vi "Set Test Method End Time.vi"(11 "LUnit Test Case in":refnum<class "LUnit Test Case.lvclass">) -> (3 "LUnit Test Case out":refnum<class "LUnit Test Case.lvclass">)   [LabVIEW 2020, in "LUnit Test Case.lvclass"]
uses:
  LUnit Test Case.lvclass
  Result Types/Case Result/Test Case Result.lvlib
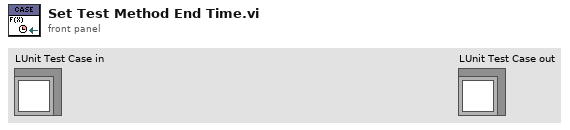
[diagram p1: front panel]
types:
  T1 = typedef "Test Case Result.lvlib/Test Case Result.ctl" = map{string, T2}
  T2 = typedef "Method Result.lvlib/Method Result.ctl" = cluster{"Test Case":string, "Test Method Name":string, "Status":T3, "Assertion Results":T4[], "Execution time":dbl, "Result String":string}
  T3 = typedef "Assertion Result.lvlib/Status.ctl" = enum16{"Pass", "Fail", "Error", "Skipped", "Setup Error", "Broken", "Teardown Error"}
  T4 = typedef "Assertion Result.lvlib/Assertion Result.ctl" = cluster{"Status":T3, "Message":string, "Description":string, "Assertion Type":T5}
  T5 = typedef "Assertion Result.lvlib/Assertion Type.ctl" = enum16{"None", "Pass", "Fail", "Skip", "Pass if Equal", "Fail if Equal", "Pass if Error", "Fail if Error", "Pass if", "Fail if"}
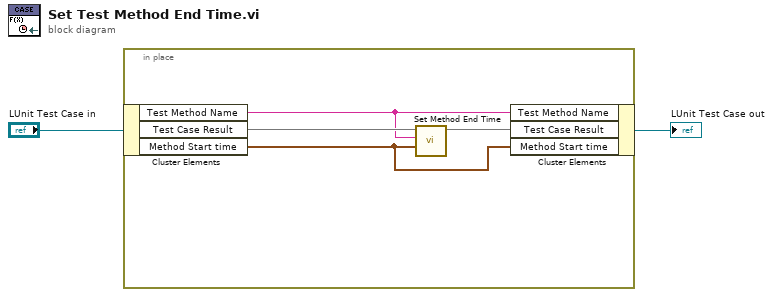
[diagram p0: block diagram]
diagram:
  n1 = in-place {
    n2 = in-place-cluster #1("LUnit Test Case in") -> ("Test Method Name"=w4:string, "Test Case Result"=w6:T1, "Method Start time"=w3:timestamp)
    n3 = call "Set Method End Time.vi"("Method Start Time"=w3, "Test Method Name"=w4, "Test Case Result In"=w6) -> ("Test Case Result Out"=w5:T1)  [unwired: 8 in]
    n4 = in-place-cluster #1("Test Method Name"=w4, "Test Case Result"=w5, "Method Start time"=w3) -> (→"LUnit Test Case out":refnum<class "LUnit Test Case.lvclass">)
  }
